vi "Update Gyro.vi"(11 "Gyro ID (1 or 2)":i32) -> ()   [LabVIEW 2013]
uses:
  Gyro Global.vi
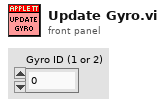
[diagram p1: front panel]
types:
  T1 = typedef "WPI_AnalogChannelDevRef.ctl" = cluster{"DevStatus":errorcluster, "Analog Module":T2, "Analog Channel":T3}
  T2 = typedef "FPGA_TypedefAnalogModule.ctl" = enum16{"Analog Module 1", "Analog Module 2"}
  T3 = typedef "FPGA_AIChannel.ctl" = enum8{"AI 1", "AI 2", "AI 3", "AI 4", "AI 5", "AI 6", "AI 7", "AI 8", "Invalid"}
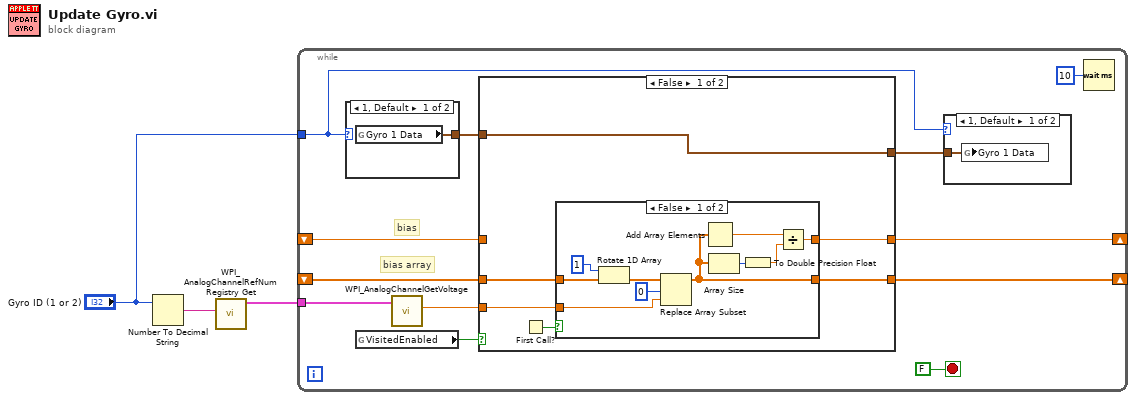
[diagram p0: block diagram]
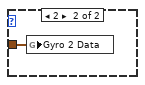
[diagram p2: hidden frame]
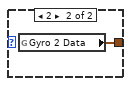
[diagram p3: hidden frame]
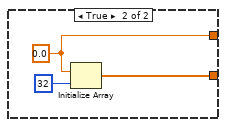
[diagram p4: hidden frame]
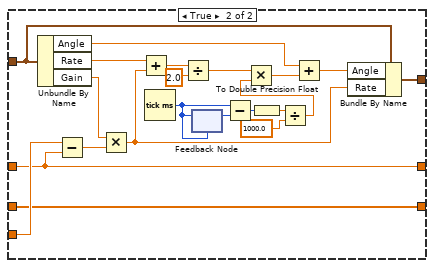
[diagram p5: hidden frame]
diagram:
  n1 = Number To Decimal String(number="Gyro ID (1 or 2)") -> (decimal integer string=w2:string)  [unwired: 1 in]
  n2 = call <vilib>:"WPI_AnalogChannelRefNum Registry Get.vi"("refnum name"=w2) -> ("AIDeviceRef"=w3:T1)  [unwired: 9 in, 1 out]
  n3 = while {
    shift-right: [w13] -> _
    shift-left: _ -> [w12]
    shift-right: [w7] -> _
    shift-left: _ -> [w10]
    tunnel: w3 -> [w9]
    tunnel: "Gyro ID (1 or 2)" -> [w4]
    stop <- FALSE stop-if-true
    # "bias"
    # "bias array"
    n4 = case shown="1, Default" w4 {
      tunnel: [w18 w19] -> w6
      frame 1, Default {
        n5 = global read "Gyro Global.vi" "Gyro 1 Data"() -> (w18:cluster{"Rate":dbl, "Angle":dbl, "Gain":dbl})
      }
      frame 2 {
        n6 = global read "Gyro Global.vi" "Gyro 2 Data"() -> (w19:cluster{"Rate":dbl, "Angle":dbl, "Gain":dbl})
      }
    }
    n7 = global read "Gyro Global.vi" "VisitedEnabled"() -> (w11:bool)
    n8 = call <vilib>:"WPI_AnalogChannelGetVoltage.vi"("AIDeviceRef"=w9) -> ("Voltage"=w8:dbl)  [unwired: 8 in, 2 out]
    n9 = case shown="False" w11 {
      tunnel: [w24 w58] -> w13
      tunnel: w12 -> [w23 w58]
      tunnel: [w22 w57] -> w7
      tunnel: w6 -> [w20 w54]
      tunnel: w8 -> [w21 w59]
      tunnel: w10 -> [_ w57]
      tunnel: [w20 w53] -> w5
      frame False {
        n10 = First Call?() -> (First Call?: T/F=w25:bool)
        n11 = case shown="False" w25 {
          tunnel: [w28 w37] -> w24
          tunnel: w23 -> [w35 _]
          tunnel: [w30 w36] -> w22
          tunnel: w21 -> [w27 _]
          frame False {
            n12 = Rotate 1D Array(1:w35, 2:1 ("n")) -> (0:w29:dbl[])
            n13 = Replace Array Subset(array=w29, new element=w27, index=0) -> (w28:dbl[])
            n14 = Add Array Elements(numeric array=w28) -> (sum=w33:dbl)
            n15 = Array Size(array=w28) -> (size(s)=w32:i32)
            n16 = To Double Precision Float(number=w32) -> (double precision float=w31:dbl)
            n17 = Divide(x=w33, y=w31) -> (x/y=w30:dbl)
          }
          frame True {
            w36 = 0.0 ("element")
            n18 = Initialize Array(w36, 32 ("dimension size")) -> (w37:dbl[])
          }
        }
      }
      frame True {
        n19 = Unbundle By Name(w54) -> ("Angle"=w40:dbl, "Rate"=w51:dbl, "Gain"=w55:dbl)
        n20 = Subtract(x=w59, y=w57) -> (x-y=w56:dbl)
        n21 = Multiply(x=w55, y=w56) -> (x*y=w52:dbl)
        n22 = Add(x=w51, y=w52) -> (x+y=w50:dbl)
        n23 = Tick Count (ms)() -> (millisecond timer value=w47:u32)
        n24 = Divide(x=w50, y=2.0) -> (x/y=w48:dbl)
        n25 = feedback-in #1(w47) -> ()
        n26 = feedback #1(w47) -> (w46:u32)
        n27 = Subtract(x=w47, y=w46) -> (x-y=w45:u32)
        n28 = To Double Precision Float(number=w45) -> (double precision float=w44:dbl)
        n29 = Divide(x=w44, y=1000.0) -> (x/y=w42:dbl)
        n30 = Multiply(x=w48, y=w42) -> (x*y=w41:dbl)
        n31 = Add(x=w40, y=w41) -> (x+y=w39:dbl)
        n32 = Bundle By Name(cluster=w54, "Angle"=w39, "Rate"=w52) -> (w53:cluster{"Rate":dbl, "Angle":dbl, "Gain":dbl})
      }
    }
    n33 = case shown="1, Default" w4 {
      tunnel: w5 -> [w16 w17]
      frame 1, Default {
        n34 = global write "Gyro Global.vi" "Gyro 1 Data"(w16) -> ()
      }
      frame 2 {
        n35 = global write "Gyro Global.vi" "Gyro 2 Data"(w17) -> ()
      }
    }
    n36 = Wait (ms)(milliseconds to wait=u32 10) -> ()  [unwired: 1 out]
  }
